vi "Matrix Inverse v1.4.vi"() -> ()   [LabVIEW 2020]
uses:
  <vilib>/Analysis/Matrix/Datatypes/RealMatrix.ctl
  <vilib>/Analysis/baseanly.llb/Mean (DBL).vi
  <vilib>/Analysis/Matrix/Numeric/Conversions/Array To Matrix - RA2.vi
  <vilib>/Analysis/baseanly.llb/Real Inverse Matrix.vi
  <vilib>/Analysis/Matrix/Numeric/Conversions/Matrix To Array - RM.vi
  <vilib>/Analysis/NI_AALBase.lvlib
  <vilib>/Analysis/Matrix/NI_Matrix.lvlib
panel:
  out "pt - pt error":sgl[][](array[numeric])
  out "percent error":dbl format="%0.2f"
  out "x > y?":bool
  out "divide by zero detected":bool
  out "A":T1
  out "sum of error":sgl
  out "inv(A) LABVIEW-FPGA":sgl[][](array[numeric])
  out "inv(A) LABVIEW":T1
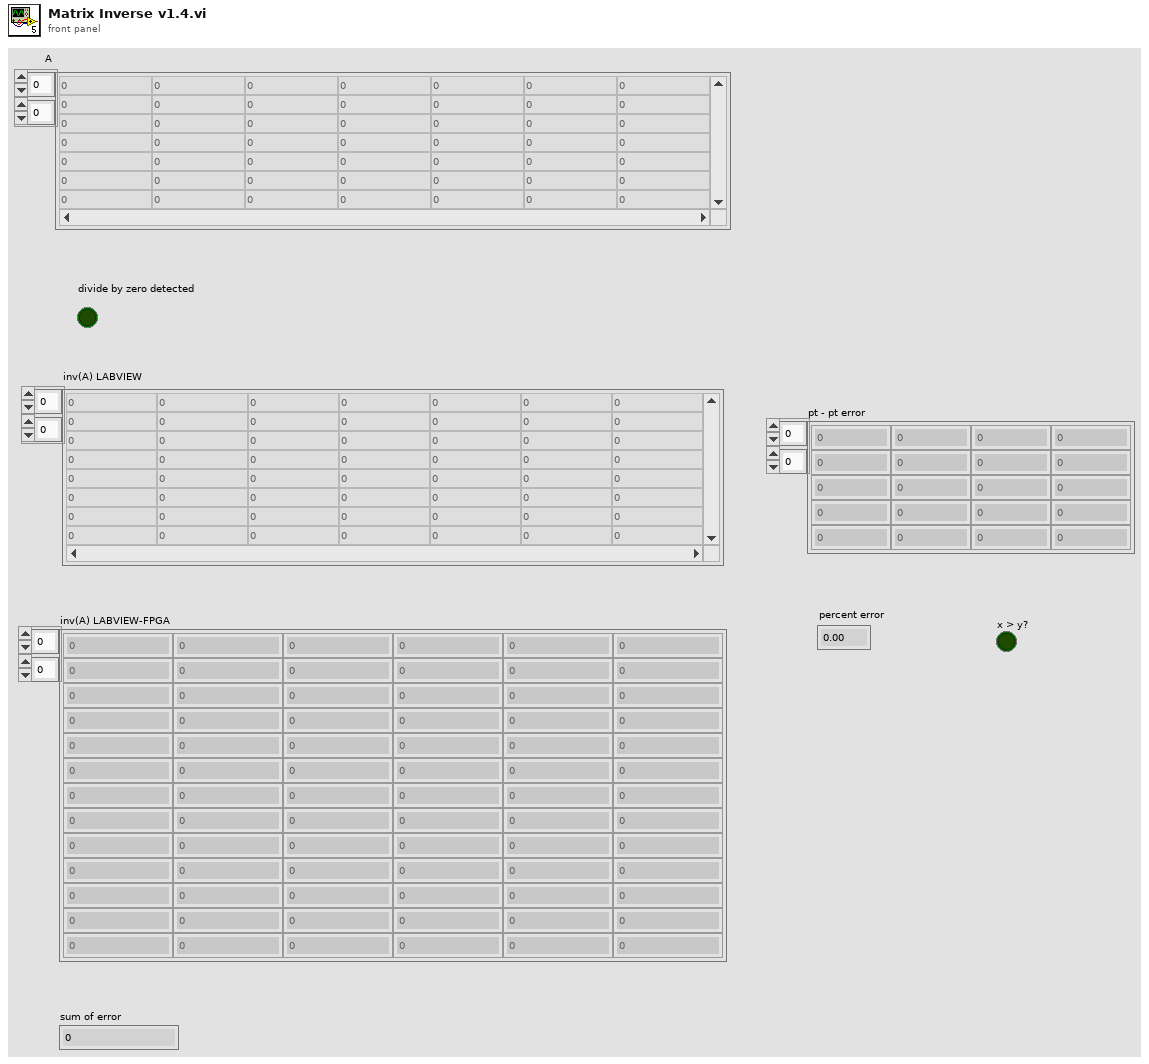
[diagram p1: front panel]
types:
  T1 = typedef "NI_Matrix.lvlib/RealMatrix.ctl" = dbl[][]
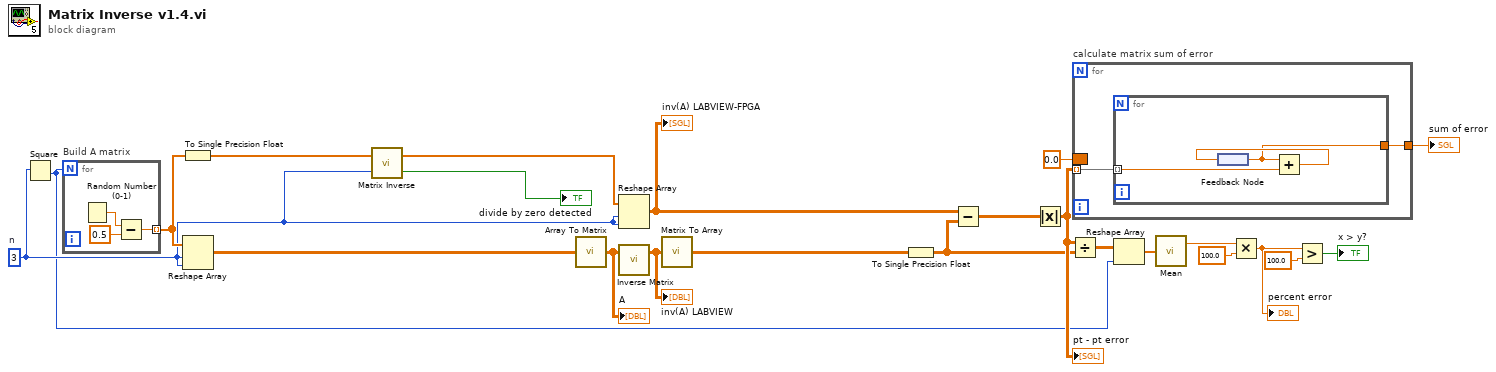
[diagram p0: block diagram]
diagram:
  w3 = 3  # n
  n1 = Square(x=w3) -> (x^2=w1:i32)
  n2 = for "Build A matrix" {
    N: w1 -> [_]
    tunnel: [w24] -> w21 mode=indexing
    n3 = Random Number (0-1)() -> (number: 0 to 1=w26:dbl)
    n4 = Subtract(x=w26, y=0.5) -> (x-y=w24:dbl)
  }
  n5 = To Single Precision Float(number=w21) -> (single precision float=w20:sgl[])
  n6 = Reshape Array(w21, w3, w3) -> (w23:dbl[][])
  n7 = call "Matrix Inverse.vi"("n"=w3, "A"=w20) -> ("divide by zero detected"=→"divide by zero detected":bool, "inv(A)"=w19:sgl[])
  n8 = call-poly <vilib>:"Array To Matrix.vi"("Real 2D Array"=w23) -> ("Real Matrix"=w22:T1)
  "A" <- w22
  n9 = Reshape Array(w19, w3, w3) -> (w12:sgl[][])
  "inv(A) LABVIEW-FPGA" <- w12
  n10 = call-poly <vilib>:"Inverse Matrix.vi"("Input Matrix"=w22) -> ("Inverse Matrix"=w17:T1)  [unwired: 1 in, 1 out]
  "inv(A) LABVIEW" <- w17
  n11 = call-poly <vilib>:"Matrix To Array.vi"("Real Matrix"=w17) -> ("Real 2D Array"=w16:dbl[][])
  n12 = To Single Precision Float(number=w16) -> (single precision float=w10:sgl[][])
  n13 = Subtract ("Subtract.vi")(x=w12, y=w10) -> (x-y=w18:sgl[][])
  n14 = Absolute Value ("Absolute Value.vi")(x=w18) -> (abs(x)=w11:sgl[][])
  "pt - pt error" <- w11
  n15 = Divide(x=w11, y=w10) -> (x/y=w9:sgl[][])
  n16 = for "calculate matrix sum of error" {
    tunnel: w11 -> [w28] mode=indexing
    tunnel: [w27] -> w15
    border: sgl 0.0 -> [_]
    n17 = for {
      tunnel: w28 -> [w31] mode=indexing
      tunnel: [w29] -> w27
      n18 = feedback #1() -> (w29:sgl)
      n19 = Add(x=w29, y=w31) -> (x+y=w30:sgl)
      n20 = feedback-in #1(w30) -> ()
    }
  }
  "sum of error" <- w15
  n21 = Reshape Array(w9, w1) -> (w8:sgl[])
  n22 = call-poly <vilib>:"Mean.vi"("X"=w8) -> ("mean"=w7:dbl)  [unwired: 1 out]
  n23 = Multiply(x=w7, y=100.0) -> (x*y=w5:dbl)
  "percent error" <- w5
  n24 = Greater?(x=w5, y=sgl 100.0) -> (0:→"x > y?":bool)
